vi "subVI_reverse_8bits.vi"(1 "8 bit number":u8) -> (0 "reversed 8 bit number":u8)   [LabVIEW 2010]
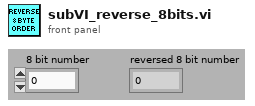
[diagram p1: front panel]
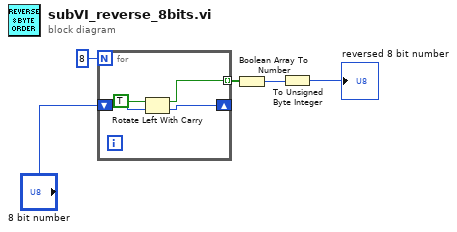
[diagram p0: block diagram]
diagram:
  n1 = for {
    N: 8 -> [_]
    shift-right: [w8] -> _
    shift-left: "8 bit number" -> [w9]
    tunnel: [w7] -> w4 mode=indexing
    n2 = Rotate Left With Carry(2:w9, 3:TRUE ("carry")) -> (0:w8:u8, 1:w7:bool)
  }
  n3 = Boolean Array To Number(Boolean array=w4) -> (number=w2:u32)
  n4 = To Unsigned Byte Integer(number=w2) -> (unsigned 8bit integer=→"reversed 8 bit number":u8)
